vi "commandURL.vi"(4 "Command String":string, 5 "Scanner IP Address":string) -> (0 "Command URL":string)   [LabVIEW 2019, in "PF_API.lvclass"]
doc: "This SubVI builds the URL of a command that can be sent to the scanner using HTTP Protocol. Use it in combination with addParameter.vi to build a command with custom parameters."
uses:
  PF_API.lvclass
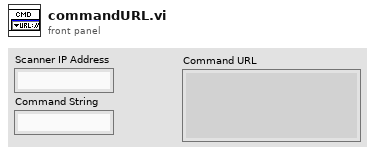
[diagram p1: front panel]
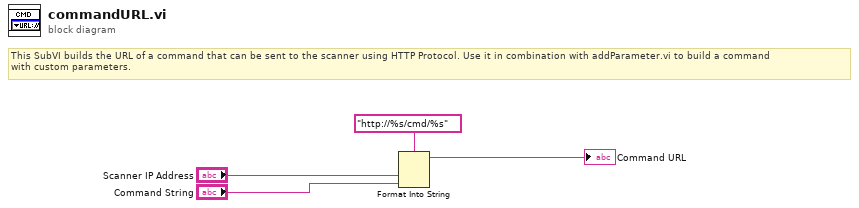
[diagram p0: block diagram]
diagram:
  # "This SubVI builds the URL of a command that can be sent to the scanner using HTTP Protocol. Use it in combination with addParameter.vi to build a command\nwith custom parameters."
  n1 = Format Into String(format string="http://%s/cmd/%s", "Scanner IP Address", "Command String") -> (resulting string=→"Command URL":string)  [unwired: 2 in, 1 out]
